vi "calibration method2.vi"(0 "session in":refnum<k35>, 1 "function name":string="fit", 5 "Image IN":T1(plugin-control), 7 "initialize matrix":dbl[][](array[numeric]), 9 "module path":path, 11 "error in":errorcluster, 12 "snap number":i32) -> (4 "session out":refnum<k35>, 8 "calibration matrix":dbl[][](array[numeric]), 15 "error out":errorcluster)   [LabVIEW 2019, in "Calibration Lib.lvlib"]
uses:
  Calibration Lib.lvlib
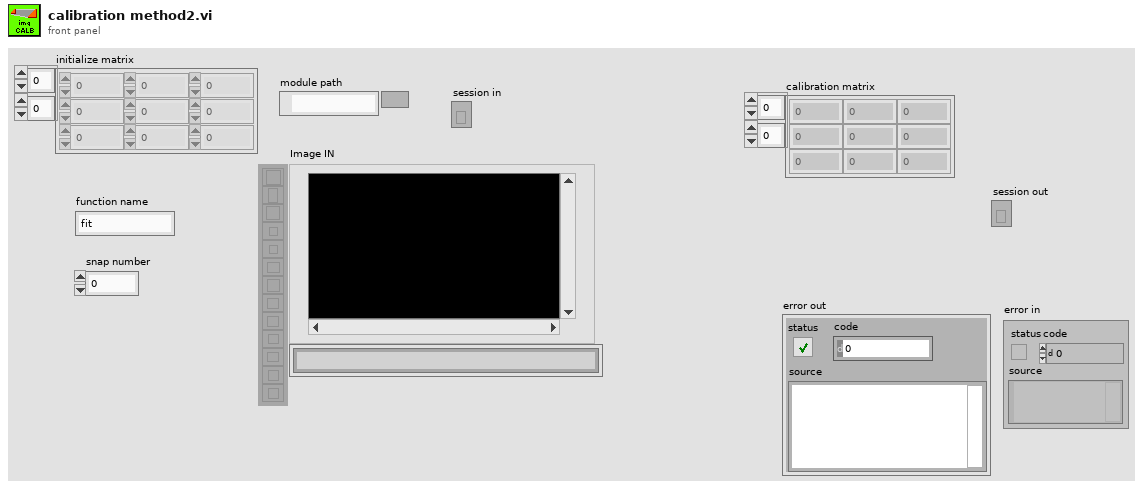
[diagram p1: front panel]
types:
  T1 = typedef "IMAQ Image.ctl" = refnum<image>
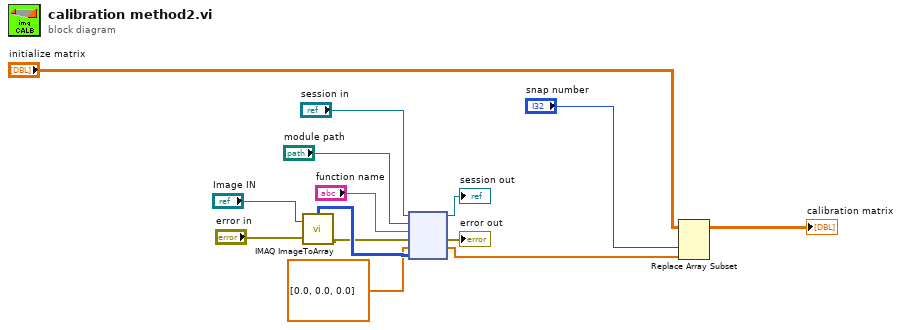
[diagram p0: block diagram]
diagram:
  n1 = call "IMAQ ImageToArray"("error in (no error)"="error in", "Image"="Image IN") -> ("error out"=w7:errorcluster, "Image Pixels (U8)"=w9:u8[][])  [unwired: 2 in, 3 out]
  n2 = node("session in", "module path", "function name", w7, dbl[] [0.0, 0.0, 0.0], w9) -> (→"session out":refnum<k35>, →"error out":errorcluster, w2:dbl[])  [unwired: 1 in, 2 out]
  n3 = Replace Array Subset(array="initialize matrix", new element=w2, index (col)="snap number") -> (→"calibration matrix":dbl[][])  [unwired: 1 in]
